vi "Single_ADC_Calc.vi"(5 "aDATA":u8[](array[numeric]), 6 "Number Of Retry In":u32, 7 "Retry Delay In":u32, 8 "On Delay  In":u32, 9 "Current TH In":u32) -> (0 "Retry Delay Out":u32, 1 "Number Of Retry Out":u32, 2 "On Delay Out":u32, 3 "Current TH Out":u32, 4 "CH R":u8)   [LabVIEW 2010]
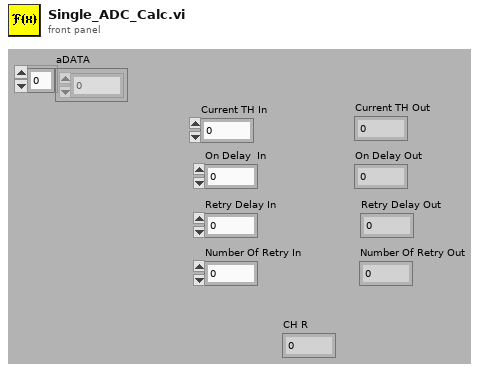
[diagram p1: front panel]
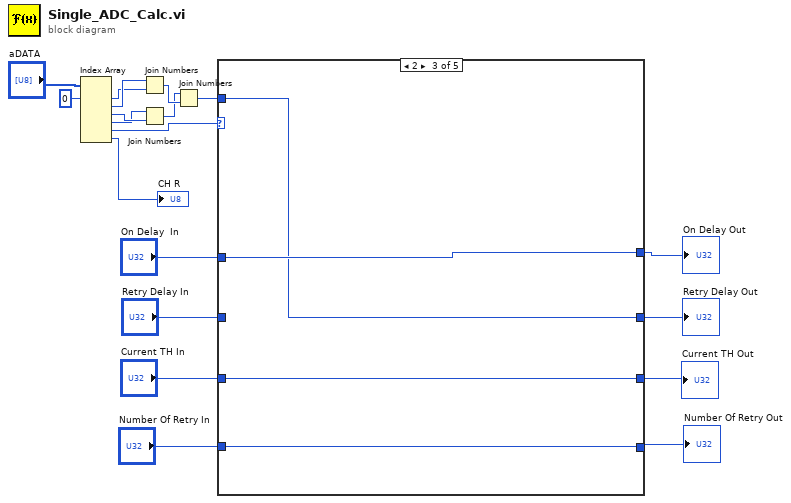
[diagram p0: block diagram]
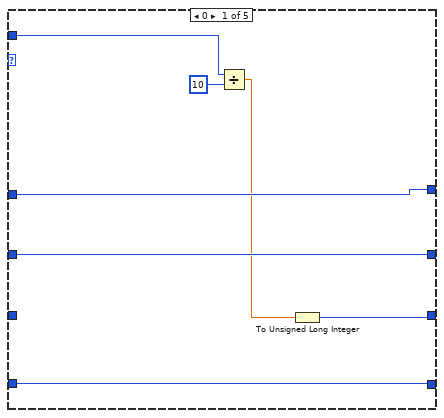
[diagram p2: hidden frame]
diagram:
  n1 = Index Array(array="aDATA", index #1=0 ("index")) -> (element #1=w13:u8, element #2=w14:u8, element #3=w16:u8, element #4=w15:u8, element #5=w2:u8, element #6=→"CH R":u8)  [unwired: 5 in]
  n2 = Join Numbers(hi=w14, lo=w13) -> ((hi.lo)=w19:u16)
  n3 = Join Numbers(hi=w15, lo=w16) -> ((hi.lo)=w18:u16)
  n4 = Join Numbers(hi=w18, lo=w19) -> ((hi.lo)=w11:u32)
  n5 = case shown="2" w2 {
    tunnel: w11 -> [w25 w30 w32 w35 _]
    tunnel: [w24 w30 w34 w38 w42] -> w10
    tunnel: "On Delay  In" -> [w24 _ w34 w38 w42]
    tunnel: "Retry Delay In" -> [w23 w28 _ w36 w40]
    tunnel: [w23 w28 w32 w36 w40] -> w7
    tunnel: "Current TH In" -> [_ w29 w33 w37 w41]
    tunnel: [w21 w29 w33 w37 w41] -> w5
    tunnel: "Number Of Retry In" -> [w20 w27 w31 _ w39]
    tunnel: [w20 w27 w31 w35 w39] -> w3
    frame 0 {
      n6 = Divide(x=w25, y=u32 10) -> (x/y=w22:dbl)
      n7 = To Unsigned Long Integer(number=w22) -> (unsigned 32bit integer=w21:u32)
    }
    frame 1 {
    }
    frame 2 {
    }
    frame 3 {
    }
    frame 4, Default {
    }
  }
  "On Delay Out" <- w10
  "Retry Delay Out" <- w7
  "Current TH Out" <- w5
  "Number Of Retry Out" <- w3
